vi "RT Main.vi"() -> ()   [LabVIEW 2021]
uses:
  <vilib>/Platform/TimedLoop/XDataNode/timing_clust.ctl
  <vilib>/Platform/TimedLoop/XDataNode/nitl_modes.ctl
  <vilib>/Platform/TimedLoop/XDataNode/wakeup.ctl
  <vilib>/myRIO/Common/Instrument Driver Framework/myRIO v1.0/UART/vis/myRIO v1.0 Close UART.vi
  <vilib>/myRIO/Common/Instrument Driver Framework/Utilities/vis/FPGA Ref Manager.vi
  <vilib>/myRIO/Common/Instrument Driver Framework/myRIO v1.0/myRIO v1.0 Reset FPGA.vi
  <vilib>/myRIO/Common/Instrument Driver Framework/myRIO v1.0/IRQ/vis/myRIO v1.0 IRQ Info FGV.vi
  <vilib>/myRIO/Common/Instrument Driver Framework/myRIO v1.0/IRQ/vis/myRIO v1.0 Timer IRQ Info FGV.vi
  <vilib>/myRIO/Common/Instrument Driver Framework/myRIO v1.0/IRQ/vis/myRIO v1.0 ISR Agent.vi
  <vilib>/myRIO/Instrument Drivers/Utilities/vis/Reset Index.vi
  <vilib>/myRIO/Common/Instrument Driver Framework/myRIO v1.0/Resource Manager/vis/myRIO v1.0 Block Write Resource Manager.vi
  <vilib>/Platform/TimedLoop/XDataNode/XDataNode.xnode
  <vilib>/Platform/TimedLoop/XDataNode/XDNodeRunTimeDep.lvlib
  <vilib>/myRIO/Instrument Drivers/Utilities/Utilities.lvlib
  <resource>/objmgr/ni.dex.rc
panel:
  out "End?":bool
  out "connected?":bool
  out "error out":errorcluster
  in  "stop":bool
  # "Overview: This example publishes data acquired from the accelerometer in myRIO, calculates rotation vector and rotation angle, and communicates with desktop based on network stream.                     \nRequirements: Network Streams on NI myRIO\nInstructions:\n1 Check the myRIO target IP Address in the project and make sure the target IP Address is correct.\n2. Run this VI."
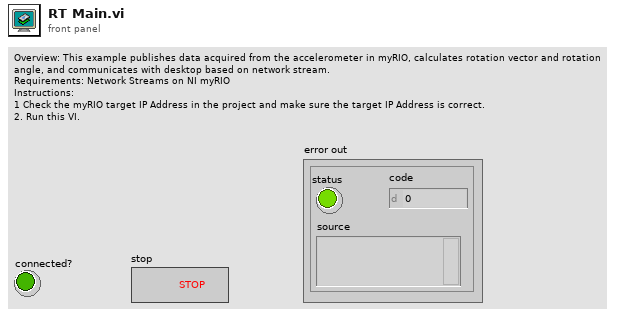
[diagram p1: front panel]
types:
  T1 = cluster{"X-Axis":dbl, "Y-Axis":dbl, "Z-Axis":dbl}
  T2 = cluster{"Numeric":dbl, "Cluster 2":cluster{"Numeric":dbl, "Numeric 2":dbl, "Numeric 3":dbl}}
  T3 = typedef "XDNodeRunTimeDep.lvlib/timing_clust.ctl" = cluster{"Expected End [f-1]":u64, "Actual End [f-1]":u64, "Finished Late? [f-1]":bool, "Expected End [i-1]":u64, "Actual End [i-1]":u64, "Finished Late? [i-1]":bool, "Expected Start [i]":u64, "Actual Start [i]":u64, "Expected Start [f]":u64, "Actual Start [f]":u64, "Source Name":string, "Structure Name":string, "Period":i64, "Deadline":i64, "Offset":i64, "Start":i64, "Priority":i32, "Timeout":i32, "Mode":T4, "Wakeup Reason":T5, "Error":errorcluster, "Source Type":string, "Secondary Source Type":string, "Global End Time":u64, "Global Start Time":u64, "Frame Duration":u64, "Iteration Duration":u64, "Assigned CPU":i32, "I/O Scan Engine Mode":u32}
  T4 = typedef "XDNodeRunTimeDep.lvlib/nitl_modes.ctl" = enum32{"No Change", "Process missed periods, maintain original phase", "Discard missed periods, maintain original phase", "Process missed periods, ignore original phase", "Discard missed periods, ignore original phase"}
  T5 = typedef "XDNodeRunTimeDep.lvlib/wakeup.ctl" = enum32{"Normal", "Aborted", "Asynchronous wakeup", "Timing source error", "Timed loop error", "Timeout"}
  T6 = typedef "Connections.ctl" = cluster{"Connections":cluster{"Ping1D - A":cluster{"Connection":refnum<visa-resource-name>, "error":errorcluster, "Distance":dbl}, "Ping1D - B":cluster{"Connection":refnum<visa-resource-name>, "error":errorcluster, "Distance":dbl}}}
  T7 = cluster{"Filtered x":dbl, "Filtered x":dbl, "Filtered x":dbl}
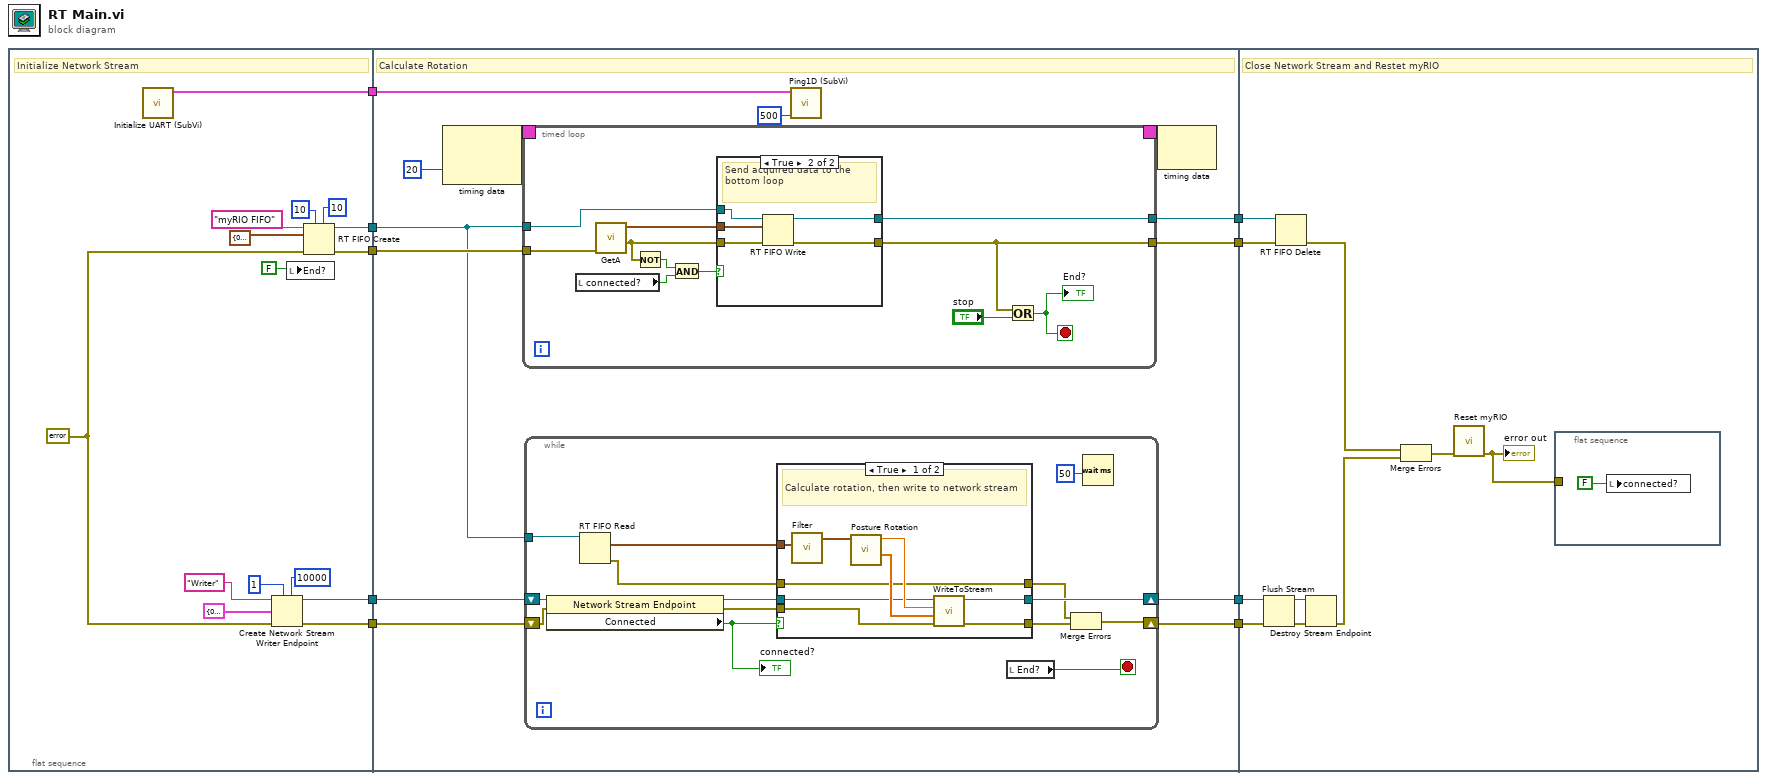
[diagram p0: block diagram]
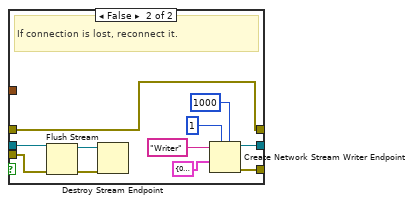
[diagram p2: hidden frame]
diagram:
  n1 = flat-sequence {
    tunnel: [w23] -> w9
    tunnel: [w22] -> w8
    tunnel: [w16] -> w5
    tunnel: [w15] -> w4
    tunnel: [w10] -> w1
    tunnel: w9 -> [w37]
    tunnel: w8 -> [w36]
    tunnel: [w35] -> w7
    tunnel: [w34] -> w6
    tunnel: w5 -> [w31]
    tunnel: w4 -> [w28]
    tunnel: [w30] -> w3
    tunnel: [w29] -> w2
    tunnel: w1 -> [w25]
    tunnel: w7 -> [w103]
    tunnel: w6 -> [w102]
    tunnel: w3 -> [w101]
    tunnel: w2 -> [w100]
    frame #0 {
      w11 = errorcluster {"status"=FALSE, "code"=0, "source"=""} ("error in (no error)")
      # "Initialize Network Stream"
      n2 = call "Initialize UART (SubVi).vi"() -> ("Connections"=w10:T6)  [unwired: 11 in]
      n3 = Create Network Stream Writer Endpoint(5:10000 ("timeout in ms (-1)"), 7:1 ("writer buffer size"), 8:w11, 9:T2 {"Numeric"=0.0, "Cluster 2"={"Numeric"=0.0, "Numeric 2"=0.0, "Numeric 3"=0.0}} ("Cluster"), 11:"Writer" ("reader url")) -> (0:w22:errorcluster, 3:w23:refnum<k21>)  [unwired: 2 in]
      n4 = local write "End?"(FALSE) -> ()
      n5 = RT FIFO Create(0:"myRIO FIFO" ("name (unnamed)"), 1:T1 {"X-Axis"=0.0, "Y-Axis"=0.0, "Z-Axis"=0.0}, 3:w11, 4:u32 10 ("size (10)"), 6:u32 10 ("elements in array (1)")) -> (8:w15:refnum<k33>, 11:w16:errorcluster)  [unwired: 3 in, 1 out]
    }
    frame #1 {
      # "Calculate Rotation"
      n6 = node-c288(i64 20 ("Period")) -> (w33:T3)  [unwired: 1 in]
      n7 = timed-loop {
        timing: w33 -> [_]
        timing-out: [_] -> w32
        tunnel: w31 -> [w82]
        tunnel: w28 -> [w79]
        tunnel: [w81] -> w30
        tunnel: [w72] -> w29
        stop <- w78 stop-if-true
        n8 = local read "connected?"() -> (w75:bool)
        n9 = call "GetA.vi"("error in (no error)"=w82) -> ("error out"=w74:errorcluster, "A"=w80:T1)  [unwired: 9 in]
        n10 = Not(x=w74) -> (.not. x?=w73:bool)
        n11 = And(x=w73, y=w75) -> (x .and. y?=w76:bool)
        n12 = case shown="True" w76 {
          tunnel: [w84 w89] -> w81
          tunnel: w80 -> [_ w87]
          tunnel: [w83 w88] -> w72
          tunnel: w79 -> [w84 w86]
          tunnel: w74 -> [w83 w85]
          frame False {
          }
          frame True {
            # "Send acquired data to the bottom loop"
            n13 = RT FIFO Write(0:w86, 1:w87, 3:w85) -> (8:w89:refnum<k33>, 11:w88:errorcluster)  [unwired: 2 in, 2 out]
          }
        }
        n14 = Or(x=w72, y="stop") -> (x .or. y?=w78:bool)
        "End?" <- w78
      }
      n15 = while {
        shift-right: [w38] -> w34
        shift-left: w36 -> [w48]
        shift-right: [w45] -> w35
        shift-left: w37 -> [w49]
        tunnel: w28 -> [w51]
        stop <- w41 stop-if-true
        n16 = property class="Network Stream Endpoint"(reference=w49, error in=w48) -> (reference out=w47:refnum<k21>, error out=w46:errorcluster, "Connected"=w43:bool)
        "connected?" <- w43
        n17 = RT FIFO Read(0:w51) -> (9:w50:T1, 11:w44:errorcluster)  [unwired: 3 in, 3 out]
        n18 = case shown="True" w43 {
          tunnel: w50 -> [w57 _]
          tunnel: w47 -> [w56 w64]
          tunnel: w46 -> [w55 w62]
          tunnel: [w54 w71] -> w45
          tunnel: [w53 w66] -> w39
          tunnel: w44 -> [w52 w65]
          tunnel: [w52 w65] -> w40
          frame True {
            # "Calculate rotation, then write to network stream"
            n19 = call "Filter.vi"("A"=w57) -> ("Low Freq. A"=w58:T7)  [unwired: 10 in]
            n20 = call "Posture Rotation.vi"("Rotation X,Y,Z"=w58) -> ("Rotation Vector"=w59:dbl[], "Rotation Angle"=w60:dbl)  [unwired: 9 in]
            n21 = call "WriteToStream.vi"("error in"=w55, "Vector"=w59, "Angle"=w60, "endpoint in"=w56) -> ("error out"=w53:errorcluster, "endpoint out"=w54:refnum<k21>)  [unwired: 6 in]
          }
          frame False {
            # "If connection is lost, reconnect it."
            n22 = Flush Stream(8:w62, 11:w64) -> (0:w61:errorcluster, 3:w63:refnum<k21>)  [unwired: 2 in, 1 out]
            n23 = Destroy Stream Endpoint(8:w61, 11:w63) -> ()  [unwired: 1 out]
            n24 = Create Network Stream Writer Endpoint(5:1000 ("timeout in ms (-1)"), 7:1 ("writer buffer size"), 9:T2 {"Numeric"=0.0, "Cluster 2"={"Numeric"=0.0, "Numeric 2"=0.0, "Numeric 3"=0.0}} ("Cluster"), 11:"Writer" ("reader url")) -> (0:w66:errorcluster, 3:w71:refnum<k21>)  [unwired: 3 in]
          }
        }
        n25 = local read "End?"() -> (w41:bool)
        n26 = Merge Errors(w40, w39) -> (w38:errorcluster)
        n27 = Wait (ms)(milliseconds to wait=50) -> ()  [unwired: 1 out]
      }
      n28 = call "Ping1D (SubVi).vi"("Comm. Delay"=u32 500, "Connections"=w25) -> ()  [unwired: 9 in, 1 out]
      n29 = node-c288(w32) -> ()  [unwired: 1 out]
    }
    frame #2 {
      # "Close Network Stream and Restet myRIO"
      n30 = Flush Stream(8:w102, 11:w103) -> (0:w105:errorcluster, 3:w104:refnum<k21>)  [unwired: 2 in, 1 out]
      n31 = RT FIFO Delete(0:w101, 3:w100) -> (11:w99:errorcluster)  [unwired: 1 in]
      n32 = Destroy Stream Endpoint(8:w105, 11:w104) -> (0:w98:errorcluster)
      n33 = Merge Errors(w99, w98) -> (w97:errorcluster)
      n34 = call <vilib>:"Reset myRIO.vi"("error in (no error)"=w97) -> ("error out"=w96:errorcluster)  [unwired: 10 in]
      "error out" <- w96
      n35 = flat-sequence {
        tunnel: w96 -> [_]
        frame #0 {
          n36 = local write "connected?"(FALSE) -> ()
        }
      }
    }
  }
